vi "TWIN_v15_5.vi"() -> ()   [LabVIEW 2017]
uses:
  BERTTA/x64/Debug/BERTTA.dll
panel:
  in  "Add comment":string
  in  "OK Button":bool
  out "Started:":string
  in  "SHUTDOWN":bool
  in  "MASTER CONTROL":bool
  in  "Tab Control":T1(tab)
  out "Output File":path caption="selected path"
  in  "Browse folder":path=path "C:/Users/shresplab/Desktop" caption="start path"
  in  "Read Seq":bool
  in  "Save Seq":bool
  in  "Configuration file":path caption="Filename"
  in  "OK Button 2":bool
  out "Boolean":bool
  in  "User (initials)":string
  in  "Project name":string
  in  "Description":string
  out "Waveform Chart 9":dynamicdata(graph)
  out "Sensor OK 10":bool
  out "Sensor OK 9":bool
  out "Sensor OK 8":bool
  out "Sensor OK 7":bool
  out "Tr 2":dbl format="Tr:              %#_4g"
  out "Tj in 2":dbl format="Tj in:        %#_4g"
  out "Tj out 2":dbl format="Tj out:        %#_4g"
  out "T set 2":dbl format="T set:          %#_4g"
  out "Current step 3":i32 format="Current step:  %.0f"
  out "RPM 6":dbl format="RPM:          %#_g"
  out "Torque 4":dbl format="Torque:      %#_g"
  out "T external 5":dbl format="T (S2):       %#_4g"
  out "PUMP3 2":bool
  out "Led11 17":bool
  out "Target amount 2":dbl
  out "Scale weight 2":dbl
  out "Amount now 3":dbl
  out "Flow rate 2":dbl
  out "Time to target 5":dbl format="%<%H:%M:%S>t"
  out "Current step 2":dbl
  out "Target 2":dbl
  out "Amount now 2":dbl
  out "Led11 12":bool
  out "Target amount":dbl
  out "Scale weight":dbl
  out "Amount now":dbl
  out "Flow rate":dbl
  out "Time to target":dbl format="%<%H:%M:%S>t"
  out "Current step":dbl
  out "Target":dbl
  out "Amount now":dbl
  out "PUMP3":bool
  out "Led11 11":bool
  out "Amount now":dbl
  out "Target":dbl
  out "Current step":dbl
  out "Time to target":dbl format="%<%H:%M:%S>t"
  out "Flow rate":dbl
  out "Amount now":dbl
  out "Scale weight":dbl
  out "Target amount":dbl
  out "PUMP2":bool
  out "Target amount":dbl format="Target amount:        %#_g"
  out "Scale weight":dbl format="Scale weight:     %#_4g"
  out "Amount now":dbl format="Amount now:      %#_4g"
  out "Flow rate":dbl format="Flow rate:                   %#_4g"
  out "Time to target":dbl format="Time to target:     %<%H:%M:%S>t"
  out "Current step":dbl format="Current step:              %#_g"
  out "Target":dbl format="Target:                %#_4g"
  out "Amount now":dbl format="Amount now:    %#_4g"
  out "Led11 10":bool
  out "PUMP1":bool
  out "Sensor OK 6":bool
  out "Sensor OK 5":bool
  out "Sensor OK 4":bool
  out "Sensor OK 3":bool
  out "Tr":dbl format="Tr:              %#_4g"
  out "Tj in":dbl format="Tj in:        %#_4g"
  out "Tj out":dbl format="Tj out:        %#_4g"
  out "T set":dbl format="T set:          %#_4g"
  out "Current step":i32 format="Current step:  %.0f"
  out "RPM":dbl format="RPM:          %#_g"
  out "Torque 2":dbl format="Torque:      %#_g"
  out "T external 3":dbl format="T (S2):       %#_4g"
  out "Waveform Chart 5":dynamicdata(graph)
  out "Waveform Chart 6":dynamicdata(graph)
  out "Waveform Chart 7":dynamicdata(graph)
  in  "OK Button 11":bool=TRUE
  out "Table":string[][](table)=[["14.8.2017 18.06.59", "0,000000", "417,670000", "-0,150000", "1,000000", "22,220000", "23,366837", "23,574959", "23,985852", "23,690000", "240,000000", "4,000000", "0,000000", "397,000000", "-397,000000", "1,000000"], ["14.8.2017 18.07.06", "0,000000", "417,640000", "-0,120000", "1,000000", "22,220000", "23,763115", "23,906257", "23,985694", "23,680000", "240,000000", "4,000000", "0,000000", "397,000000", "-397,000000", "1,000000"], ["14.8.2017 18.07.13", "0,000000", "417,640000", "-0,120000", "1,000000", "22,220000", "23,965922", "24,013440", "23,984906", "23,670000", "240,000000", "4,100000", "3,000000", "397,000000", "-397,000000", "1,000000"], ["14.8.2017 18.07.21", "0,000000", "417,640000", "-0,120000", "1,000000", "22,220000", "23,943860", "23,900110", "23,987113", "23,670000", "240,000000", "4,000000", "0,000000", "397,000000", "-397,000000", "1,000000"], ["14.8.2017 18.07.28", "0,000000", "417,640000", "-0,120000", "1,000000", "22,220000", "23,736328", "23,600018", "23,989004", "23,660000", "240,000000", "4,000000", "0,000000", "397,000000", "-397,000000", "1,000000"], ["14.8.2017 18.07.36", "0,000000", "417,640000", "-0,120000", "1,000000", "22,220000", "23,480910", "23,324538", "23,991053", "23,660000", "240,000000", "4,000000", "0,000000", "397,000000", "-397,000000", "1,000000"], ["14.8.2017 18.07.43", "0,000000", "417,640000", "-0,120000", "2,000000", "22,220000", "23,195579", "23,008270", "23,999093", "23,650000", "240,000000", "4,000000", "0,000000", "397,000000", "-397,000000", "1,000000"], ["14.8.2017 18.07.51", "0,000000", "417,650000", "-417,650000", "1,000000", "22,220000", "22,862541", "22,649021", "24,003979", "23,650000", "240,000000", "4,000000", "0,000000", "397,000000", "-397,000000", "2,000000"], ["14.8.2017 18.07.58", "0,000000", "417,640000", "0,010000", "1,000000", "22,220000", "22,541353", "22,354878", "24,005398", "23,650000", "240,000000", "4,000000", "0,000000", "397,000000", "-397,000000", "1,000000"], ["14.8.2017 18.08.06", "0,000000", "417,640000", "0,010000", "1,000000", "22,220000", "22,347931", "22,253738", "24,007605", "23,640000", "240,000000", "4,100000", "0,000000", "397,000000", "-397,000000", "1,000000"], ["14.8.2017 18.08.13", "0,000000", "417,640000", "0,010000", "1,000000", "22,220000", "22,329030", "22,302102", "24,006028", "23,640000", "240,000000", "4,000000", "0,000000", "395,820000", "-395,820000", "1,000000"], ["14.8.2017 18.08.20", "0,000000", "417,640000", "0,010000", "1,000000", "22,220000", "22,466849", "22,511320", "24,002403", "23,630000", "240,000000", "4,000000", "0,000000", "395,830000", "-0,010000", "1,000000"], ["14.8.2017 18.08.28", "0,000000", "417,640000", "0,010000", "1,000000", "22,220000", "22,707062", "22,835101", "24,000984", "23,620000", "240,000000", "4,000000", "0,000000", "395,830000", "-0,010000", "1,000000"], ["14.8.2017 18.08.35", "0,000000", "417,640000", "0,010000", "1,000000", "22,220000", "23,054104", "23,232979", "24,001299", "23,600000", "240,000000", "4,000000", "0,000000", "395,830000", "-0,010000", "1,000000"], ["14.8.2017 18.08.43", "0,000000", "417,640000", "0,010000", "1,000000", "22,220000", "23,412371", "23,522793", "24,002560", "23,590000", "240,000000", "4,000000", "0,000000", "395,820000", "0,000000", "1,000000"], ["14.8.2017 18.08.51", "0,000000", "417,640000", "0,010000", "1,000000", "22,220000", "23,596247", "23,656125", "24,003821", "23,580000", "240,000000", "4,000000", "0,000000", "395,820000", "0,000000", "1,000000"]]
  out "LED_5 2":bool
  out "LED_4 2":bool
  in  "PAUSE/RUN 11":bool
  in  "TEMP RAMP 2":dbl[][](array[numeric])
  out "LED_3 2":bool
  out "LED_2 2":bool
  out "LED_1 2":bool
  out "LED_MANUAL 2":bool
  in  "Reset 9":bool
  in  "Manual/Ramp 2":bool=TRUE
  in  "Sensor selector 2":bool=TRUE
  in  "Tr/Tj mode selector 2":bool=TRUE
  out "LED STOP 2":bool
  in  "Failsafe 2":dbl=20.0 format="Failsafe temperature:            %#_g"
  out "Current temp 2":dbl format="Current temperature S1:       %#_4g"
  out "Sensor OK 2":bool
  out "T external 4":dbl format="Current temperature S2:       %#_4g"
  in  "OK Button 10":bool
  out "Waveform Chart 2":dynamicdata(graph)
  out "LED_5":bool
  out "LED_4":bool
  in  "PAUSE/RUN 4":bool
  in  "TEMP RAMP":dbl[][](array[numeric])
  out "LED_3":bool
  out "LED_2":bool
  out "LED_1":bool
  out "LED_MANUAL":bool
  in  "Reset 6":bool
  in  "Manual/Ramp":bool=TRUE
  in  "Sensor selector":bool=TRUE
  in  "Tr/Tj mode selector":bool=TRUE
  out "LED STOP":bool
  in  "Failsafe":dbl=20.0 format="Failsafe temperature:            %#_g"
  out "Current temp":dbl format="Current temperature S1:       %#_4g"
  out "Sensor OK":bool
  out "T external 2":dbl format="Current temperature S2:       %#_4g"
  in  "OK Button 3":bool
  out "Waveform Chart":dynamicdata(graph)
  in  "X scales":i64(slide)=50 scale=0.0..100.0
  out "Waveform Chart 19":dynamicdata(graph)
  in  "CLEAR":bool
  in  "ENABLE":bool=TRUE
  out "Led11 16":bool
  out "Led11 15":bool
  in  "PAUSE/RUN 12":bool
  in  "Tube select 4":u32(ring) items=["Big tube", "Double big tube", "Medium tube", "Small tube"]
  in  "Reset 10":bool
  out "Led11 14":bool
  in  "?":bool
  in  "Grams / min 4":dbl
  out "RPM 5":dbl format="%_4f"
  out "Flow rate (g/min) 4":dbl
  out "Scale reading 4":dbl
  out "Step amount now 4":dbl
  out "Total amount now 4":dbl
  out "Elapsed / step 4":dbl format="%<%H:%M:%S>t"
  out "Time to target 4":dbl format="%<%H:%M:%S>t"
  out "Led5 6":bool
  out "Led4 7":bool
  out "Led3 6":bool
  out "Led2 6":bool
  out "Led1 6":bool
  in  "PumpSeq 7":dbl[][](array[numeric])=[[0.0, 0.0, 0.0, 0.0, 0.0, 0.0, 0.0, 0.0, 0.0, 0.0], [0.0, 0.0, 0.0, 0.0, 0.0, 0.0, 0.0, 0.0, 0.0, 0.0], [0.0, 0.0, 0.0, 0.0, 0.0, 0.0, 0.0, 0.0, 0.0, 0.0], [0.0, 0.0, 0.0, 0.0, 0.0, 0.0, 0.0, 0.0, 0.0, 0.0], [0.0, 0.0, 0.0, 0.0, 0.0, 0.0, 0.0, 0.0, 0.0, 0.0], [0.0, 0.0, 0.0, 0.0, 0.0, 0.0, 0.0, 0.0, 0.0, 0.0], [0.0, 0.0, 0.0, 0.0, 0.0, 0.0, 0.0, 0.0, 0.0, 0.0], [0.0, 0.0, 0.0, 0.0, 0.0, 0.0, 0.0, 0.0, 0.0, 0.0], [0.0, 0.0, 0.0, 0.0, 0.0, 0.0, 0.0, 0.0, 0.0, 0.0], [0.0, 0.0, 0.0, 0.0, 0.0, 0.0, 0.0, 0.0, 0.0, 0.0]]
  out "Led11 13":bool
  in  "PAUSE/RUN 9":bool=TRUE
  out "Led11 7":bool
  out "Led11 6":bool
  in  "PAUSE/RUN 3":bool
  in  "Tube select 3":u32(ring) items=["Big tube", "Double big tube", "Medium tube", "Small tube"]
  in  "Reset 8":bool
  out "Led11 9":bool
  in  "?":bool
  in  "Grams / min 3":dbl
  out "RPM 3":dbl format="%_4f"
  out "Flow rate (g/min) 3":dbl
  out "Scale reading 3":dbl
  out "Step amount now 3":dbl
  out "Total amount now 3":dbl
  out "Elapsed / step 3":dbl format="%<%H:%M:%S>t"
  out "Time to target 3":dbl format="%<%H:%M:%S>t"
  out "Led5 5":bool
  out "Led4 5":bool
  out "Led3 5":bool
  out "Led2 5":bool
  out "Led1 5":bool
  in  "PumpSeq 6":dbl[][](array[numeric])=[[0.0, 0.0, 0.0, 0.0, 0.0, 0.0, 0.0, 0.0, 0.0, 0.0], [0.0, 0.0, 0.0, 0.0, 0.0, 0.0, 0.0, 0.0, 0.0, 0.0], [0.0, 0.0, 0.0, 0.0, 0.0, 0.0, 0.0, 0.0, 0.0, 0.0], [0.0, 0.0, 0.0, 0.0, 0.0, 0.0, 0.0, 0.0, 0.0, 0.0], [0.0, 0.0, 0.0, 0.0, 0.0, 0.0, 0.0, 0.0, 0.0, 0.0], [0.0, 0.0, 0.0, 0.0, 0.0, 0.0, 0.0, 0.0, 0.0, 0.0], [0.0, 0.0, 0.0, 0.0, 0.0, 0.0, 0.0, 0.0, 0.0, 0.0], [0.0, 0.0, 0.0, 0.0, 0.0, 0.0, 0.0, 0.0, 0.0, 0.0], [0.0, 0.0, 0.0, 0.0, 0.0, 0.0, 0.0, 0.0, 0.0, 0.0], [0.0, 0.0, 0.0, 0.0, 0.0, 0.0, 0.0, 0.0, 0.0, 0.0]]
  out "Led11 8":bool
  in  "PAUSE/RUN 8":bool=TRUE
  out "Led11 7":bool
  out "Led11 6":bool
  in  "PAUSE/RUN 2":bool
  in  "Tube select 2":u32(ring) items=["Big tube", "Double big tube", "Medium tube", "Small tube"]
  out "Led11 7":bool
  in  "?":bool
  in  "Grams / min 2":dbl
  out "RPM 2":dbl format="%_4f"
  out "Flow rate (g/min) 2":dbl
  out "Scale reading 2":dbl
  out "Step amount now 2":dbl
  out "Total amount now 2":dbl
  out "Elapsed / step 2":dbl format="%<%H:%M:%S>t"
  out "Time to target 2":dbl format="%<%H:%M:%S>t"
  out "Led5 4":bool
  out "Led4 4":bool
  out "Led3 4":bool
  out "Led2 4":bool
  out "Led1 4":bool
  in  "PumpSeq 5":dbl[][](array[numeric])=[[0.0, 0.0, 0.0, 0.0, 0.0, 0.0, 0.0, 0.0, 0.0, 0.0], [0.0, 0.0, 0.0, 0.0, 0.0, 0.0, 0.0, 0.0, 0.0, 0.0], [0.0, 0.0, 0.0, 0.0, 0.0, 0.0, 0.0, 0.0, 0.0, 0.0], [0.0, 0.0, 0.0, 0.0, 0.0, 0.0, 0.0, 0.0, 0.0, 0.0], [0.0, 0.0, 0.0, 0.0, 0.0, 0.0, 0.0, 0.0, 0.0, 0.0], [0.0, 0.0, 0.0, 0.0, 0.0, 0.0, 0.0, 0.0, 0.0, 0.0], [0.0, 0.0, 0.0, 0.0, 0.0, 0.0, 0.0, 0.0, 0.0, 0.0], [0.0, 0.0, 0.0, 0.0, 0.0, 0.0, 0.0, 0.0, 0.0, 0.0], [0.0, 0.0, 0.0, 0.0, 0.0, 0.0, 0.0, 0.0, 0.0, 0.0], [0.0, 0.0, 0.0, 0.0, 0.0, 0.0, 0.0, 0.0, 0.0, 0.0]]
  out "Led11 6":bool
  in  "Reset 7":bool
  in  "PAUSE/RUN 7":bool=TRUE
  out "Led5 7":bool
  out "Led4 6":bool
  in  "PAUSE/RUN":bool
  in  "Tube select":u32(ring) items=["Big tube", "Double big tube", "Medium tube", "Small tube"]
  out "Led11 5":bool
  out "RPM":dbl format="RPM                      %_4f"
  out "Flow rate (g/min)":dbl format="Flow rate               %#_g"
  out "Scale reading":dbl format="Scale reading       %#_g"
  out "Step amount now":dbl format="Step amount       %#_g"
  out "Total amount now":dbl format="Total amount      %#_g"
  out "Elapsed / step":dbl format="Elapsed / step      %<%H:%M:%S>t"
  out "Time to target":dbl format="Time to target     %<%H:%M:%S>t"
  out "Led5 3":bool
  out "Led4 3":bool
  out "Led3 3":bool
  out "Led2 3":bool
  out "Led1 3":bool
  in  "PumpSeq 4":dbl[][](array[numeric])=[[0.0, 0.0, 0.0, 0.0, 0.0, 0.0, 0.0, 0.0, 0.0, 0.0], [0.0, 0.0, 0.0, 0.0, 0.0, 0.0, 0.0, 0.0, 0.0, 0.0], [0.0, 0.0, 0.0, 0.0, 0.0, 0.0, 0.0, 0.0, 0.0, 0.0], [0.0, 0.0, 0.0, 0.0, 0.0, 0.0, 0.0, 0.0, 0.0, 0.0], [0.0, 0.0, 0.0, 0.0, 0.0, 0.0, 0.0, 0.0, 0.0, 0.0], [0.0, 0.0, 0.0, 0.0, 0.0, 0.0, 0.0, 0.0, 0.0, 0.0], [0.0, 0.0, 0.0, 0.0, 0.0, 0.0, 0.0, 0.0, 0.0, 0.0], [0.0, 0.0, 0.0, 0.0, 0.0, 0.0, 0.0, 0.0, 0.0, 0.0], [0.0, 0.0, 0.0, 0.0, 0.0, 0.0, 0.0, 0.0, 0.0, 0.0], [0.0, 0.0, 0.0, 0.0, 0.0, 0.0, 0.0, 0.0, 0.0, 0.0]]
  in  "?":bool
  in  "Grams / min":dbl format="Manual g/min:  %#_g"
  out "Led11 4":bool
  in  "Reset 5":bool
  out "Waveform Chart 18":dynamicdata(graph)
  in  "OK Button 4":bool
  out "Waveform Chart 16":dynamicdata(graph)
  in  "OK Button 5":bool
  out "Waveform Chart 17":dynamicdata(graph)
  in  "OK Button 6":bool
  in  "PAUSE/RUN 5":bool
  in  "?":bool
  in  "Scale port":dbl=5.0
  out "Waveform Chart 15":dynamicdata(graph)
  in  "OK Button 8":bool
  in  "PAUSE/RUN 10":bool
  in  "Set RPM 2":i32
  in  "Remote / Manual 2":bool
  out "RPM 4":dbl
  out "Torque 3":dbl
  out "Waveform Chart 8":dynamicdata(graph)
  in  "OK Button 9":bool
  in  "PAUSE/RUN 6":bool
  in  "Set RPM":i32
  in  "Remote / Manual":bool
  out "RPM":dbl
  out "Torque":dbl
  out "Waveform Chart 4":dynamicdata(graph)
  in  "OK Button 7":bool
  in  "CDAQ 1 Temp Control 2":tag="EASY9217_2"
  in  "PORT PUMP3 2":i32 format="PUMP 4 PORT:  %.0f"
  in  "SCALE 4":i32 format="SCALE 4 PORT:  %.0f"
  in  "HEIDOLPH 2":i32=3 format="HEIDOLPH 2 PORT:  %.0f"
  in  "LAUDA 2":i32=2 format="LAUDA 2 PORT:  %.0f"
  in  "CDAQ 1 Temp Control":tag="EASY9217_1"
  in  "CDAQ PAM Control":tag="EASY9747"
  in  "PORT PUMP2":i32 format="PUMP 2 PORT:  %.0f"
  in  "PORT PUMP3":i32 format="PUMP 3 PORT:  %.0f"
  in  "PORT PUMP1":i32 format="PUMP 1 PORT:  %.0f"
  in  "Save PortDev":bool
  in  "LAUDA":i32 format="LAUDA 1 PORT:  %.0f"
  in  "HEIDOLPH":i32 format="HEIDOLPH 1 PORT:  %.0f"
  in  "SCALE1":i32 format="SCALE 1 PORT:  %.0f"
  in  "SCALE2":i32 format="SCALE 2 PORT:  %.0f"
  in  "SCALE 3":i32 format="SCALE 3 PORT:  %.0f"
  # "Sensor:"
  # "Control:"
  # "Sensor:"
  # "Control:"
  # "PUMP & SCALE 4"
  # "STEP"
  # "TOTAL"
  # "PUMP & SCALE 3"
  # "STEP"
  # "TOTAL"
  # "PUMP & SCALE 2"
  # "STEP"
  # "TOTAL"
  # "PUMP & SCALE 1"
  # "STEP"
  # "TOTAL"
  # "MANUAL"
  # "RAMP"
  # "Temp Target       Time Target          Wait Time"
  # "STOP"
  # "MANUAL"
  # "RAMP"
  # "Temp Target       Time Target          Wait Time"
  # "STOP"
  # "g              min"
  # "g              min"
  # "g              min"
  # "g              min"
  # "PAM control"
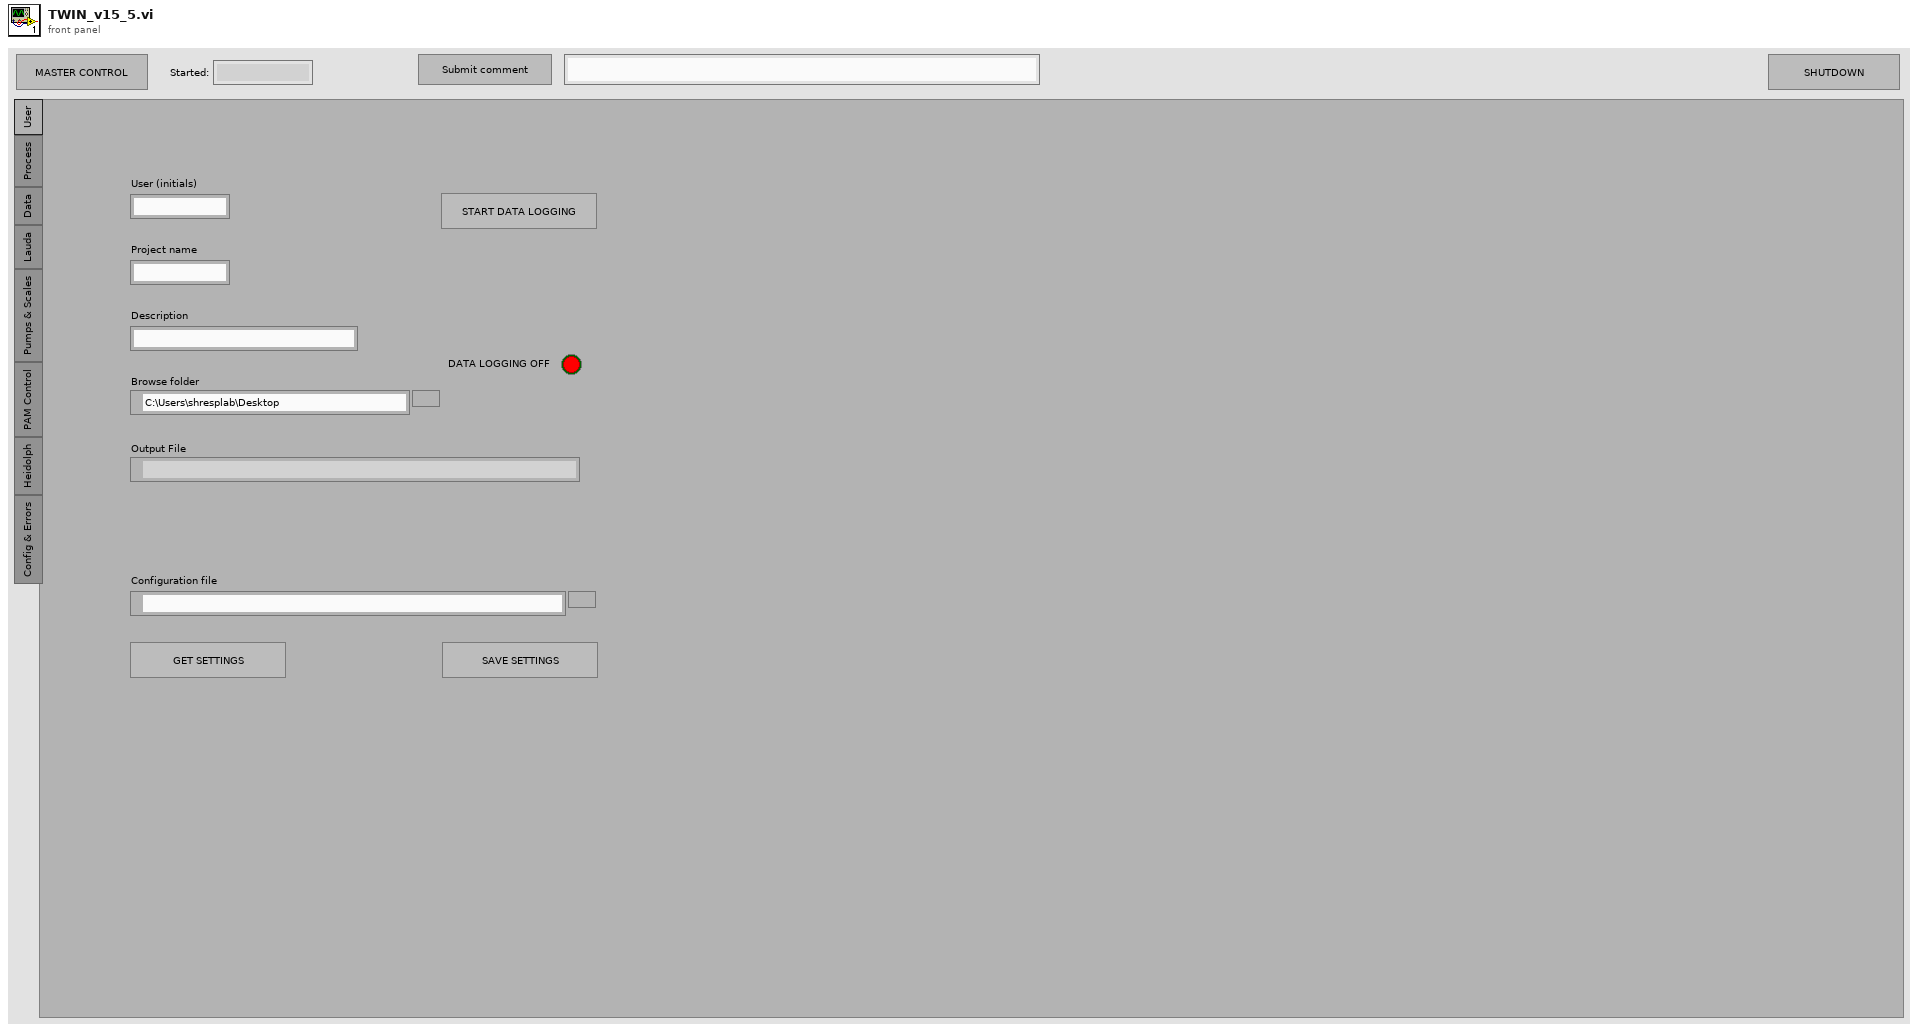
[diagram p1: front panel]
types:
  T1 = enum32{"User", "Process", "Data", "Lauda", "Pumps & Scales", "PAM Control", "Heidolph", "Config & Errors"}
diagram:
  n1 = while {
    i -> [w291]
    stop <- FALSE stop-if-true
    w225 = i64 1000 ("y")
    # "SCALE & PUMP 3"
    n2 = And(x="PAUSE/RUN 10", y="MASTER CONTROL") -> (x .and. y?=w75:bool)
    n3 = And(x="PAUSE/RUN 6", y="MASTER CONTROL") -> (x .and. y?=w215:bool)
    n4 = Not(x="MASTER CONTROL") -> (.not. x?=w326:bool)
    n5 = Boolean To (0,1)(Boolean="PAUSE/RUN 7") -> (0, 1=w4:i16)
    n6 = Boolean To (0,1)(Boolean="PAUSE/RUN 8") -> (0, 1=w3:i16)
    n7 = Boolean To (0,1)(Boolean="PAUSE/RUN 9") -> (0, 1=w2:i16)
    n8 = Boolean To (0,1)(Boolean="ENABLE") -> (0, 1=w1:i16)
    n9 = control-ref of="This VI"() -> (w211:refnum<vi>)
    n10 = Multiply(x="X scales", y=w225) -> (x*y=w226:i64)
    n11 = Boolean To (0,1)(Boolean=w326) -> (0, 1=w327:i16)
    n12 = call "RampCTRL_1.vi"("TEMP RAMP"="TEMP RAMP", "Reset 6"="Reset 6") -> ("Array"=w248:dbl[], "Array 2"=w249:dbl[], "Array 3"=w250:dbl[])  [unwired: 7 in]
    n13 = Add(x=w226, y=w225) -> (x+y=w63:i64)
    n14 = for {
      N: w327 -> [_]
      n15 = Get Date/Time String(want seconds? (F)=TRUE) -> (time string=→"Started:":string)  [unwired: 2 in, 1 out]
    }
    n16 = Select(t="Set RPM", s=w215, f=10) -> (s? t:f=w218:i32)
    n17 = Select(t="Set RPM 2", s=w75, f=10) -> (s? t:f=w72:i32)
    n18 = Boolean To (0,1)(Boolean="Sensor selector") -> (0, 1=w243:i16)
    n19 = feedback #1() -> (w224:i64)  [unwired: 1 in]
    n20 = feedback-in #1(w63) -> ()
    n21 = call "shutdown sequence.vi"("SHUTDOWN"="SHUTDOWN", "VI in"=w211) -> ()  [unwired: 10 in]
    n22 = Boolean To (0,1)(Boolean="SHUTDOWN") -> (0, 1=w210:i16)
    n23 = Boolean To (0,1)(Boolean="Reset 6") -> (0, 1=w260:i16)
    n24 = property on="Waveform Chart 2" class="WFChart (strict)"() -> ("History Data"=w65:dynamicdata[])  [unwired: 2 in, 2 out]
    n25 = Not Equal?(x=w224, y=w63) -> (x != y?=w223:bool)
    n26 = property on="Waveform Chart" class="WFChart (strict)"() -> ("History Data"=w228:dynamicdata[])  [unwired: 2 in, 2 out]
    n27 = Boolean To (0,1)(Boolean="SHUTDOWN") -> (0, 1=w212:i16)
    n28 = call "ReadMoxa12.vi"("PORT 1"="LAUDA", "PORT 2"="LAUDA 2", "PORT 3"="HEIDOLPH", "PORT 4"="HEIDOLPH 2", "PORT 5"="SCALE1", "PORT 6"="SCALE2", "PORT 7"="SCALE 3", "PORT 8"="SCALE 4", "enable1"=w4, "enable2"=w3, "enable3"=w2, "enable4"=w1) -> ("params"=w49:dbl[])  [unwired: 7 in]
    n29 = Boolean To (0,1)(Boolean=w223) -> (0, 1=w221:i16)
    n30 = Array Size(array=w228) -> (size(s)=w222:i32)
    n31 = Array Size(array=w65) -> (size(s)=w64:i32)
    n32 = call "HEI_CTRL.vi"("shutdown"=w212, "Set RPM"=w218, "Remote / Manual"="Remote / Manual", "port3"="HEIDOLPH") -> ()  [unwired: 8 in]
    n33 = Boolean To (0,1)(Boolean="Tr/Tj mode selector") -> (0, 1=w244:i16)
    n34 = call "SensorMode1.vi"("Numeric"=w243, "Numeric 2"=w244) -> ("Sensor OK 4"=→"Sensor OK 4":bool, "Sensor OK 5"=→"Sensor OK 5":bool, "Sensor OK 6"=→"Sensor OK 6":bool, "Sensor OK 3"=→"Sensor OK 3":bool)  [unwired: 6 in]
    n35 = for {
      N: w221 -> [_]
      tunnel: w222 -> [w346]
      tunnel: w63 -> [w345]
      tunnel: w64 -> [w342]
      tunnel: w63 -> [w341]
      n36 = Add(x=w342, y=w341) -> (x+y=w343:i64)
      n37 = Add(x=w346, y=w345) -> (x+y=w344:i64)
      n38 = property on="Waveform Chart" class="WFChart (strict)"("XScale.Maximum"=w344) -> ()  [unwired: 2 in, 2 out]
      n39 = property on="Waveform Chart 2" class="WFChart (strict)"("XScale.Maximum"=w343) -> ()  [unwired: 2 in, 2 out]
    }
    n40 = Boolean To (0,1)(Boolean="Manual/Ramp") -> (0, 1=w258:i16)
    n41 = And(x="MASTER CONTROL", y="PAUSE/RUN 4") -> (x .and. y?=w257:bool)
    n42 = Build Array("LAUDA", "LAUDA 2", "HEIDOLPH", "HEIDOLPH 2", "SCALE1", "SCALE2", "SCALE 3", "SCALE 4", "PORT PUMP1", "PORT PUMP2", "PORT PUMP3", "PORT PUMP3 2") -> (w232:i32[])
    n43 = Boolean To (0,1)(Boolean=w257) -> (0, 1=w256:i16)
    n44 = Boolean To (0,1)(Boolean="SHUTDOWN") -> (0, 1=w70:i16)
    n45 = call "LaudaDAQ.vi"("device name"="CDAQ 1 Temp Control") -> (1:"Tj out"=→"Tj out":dbl, "data"=w320:dynamicdata, "Sensor OK"=→"Sensor OK":bool, 4:"Tj out"=→"Tj in":dbl, "T external 2"=w214:dbl)  [unwired: 5 in, 1 out]
    "T external 2" <- w214
    "T external 3" <- w214
    n46 = call "Ramp_Lauda_v3.vi"("manual"=w258, "Tr_Tj"=w244, "shutdown"=w210, "S1_S2"=w243, "Tr"=w49, "T_fail"="Failsafe", "enable"=w256, "time_set"=w249, "reset"=w260, "time_wait"=w248, "T_S2"=w214, "port"="LAUDA", "T_sp"=w250) -> ("LED_1"=→"LED_1":bool, "LED_manual"=→"LED_MANUAL":bool, "LED_2"=→"LED_2":bool, "step"=w235:dbl, "LED_stop"=→"LED STOP":bool, "LED_3"=→"LED_3":bool, "LED 4"=→"LED_4":bool, "LED 5"=→"LED_5":bool, "setpoint"=w8:dbl, "Tr_out"=w255:dbl, "T int"=w254:dbl)  [unwired: 2 in, 2 out]
    "Tr" <- w255
    "T set" <- w8
    "Current temp" <- w255
    n47 = call "HEI_CTRL_2.vi"("shutdown"=w70, "Set RPM"=w72, "Remote / Manual"="Remote / Manual 2", "port3"="HEIDOLPH 2") -> ()  [unwired: 8 in]
    n48 = Boolean To (0,1)(Boolean="Save PortDev") -> (0, 1=w294:i16)
    n49 = for {
      N: w294 -> [_]
      tunnel: w232 -> [w400]
      tunnel: "Save PortDev" -> [w401]
      n50 = call "Convert to Dynamic Data"("Array"=w400) -> ("Dynamic Data Type"=w399:dynamicdata)  [unwired: 3 in]
      n51 = call "Write To Measurement File3"("Signals"=w399, "Reset"=w401) -> ()  [unwired: 15 in, 3 out]
    }
    n52 = Boolean To (0,1)(Boolean="OK Button 9") -> (0, 1=w67:i16)
    n53 = for {
      N: w67 -> [_]
      n54 = property on="Waveform Chart 8" class="WFChart (strict)"("History Data"=dynamicdata[] []) -> ()  [unwired: 2 in, 2 out]
    }
    n55 = Add(x=w235, y=1.0) -> (x+y=→"Current step":dbl)
    n56 = Merge Signals(w8, w255, w254, w320) -> (w22:dynamicdata)
    "Waveform Chart" <- w22
    "Waveform Chart 5" <- w22
    n57 = Less?(x=w291, y=1.0) -> (x < y?=w289:bool)
    n58 = call "HEI_Data.vi"("params"=w49) -> ("Waveform Chart 8"=→"Waveform Chart 8":dynamicdata, "RPM"=→"RPM":dbl, "Dynamic Data"=w44:dynamicdata, "RPM 2"=→"RPM":dbl, "RPM 6"=→"RPM 6":dbl, "Torque 4"=→"Torque 4":dbl, "Torque 2"=→"Torque 2":dbl, "Waveform Chart 4"=→"Waveform Chart 4":dynamicdata, "Torque 3"=→"Torque 3":dbl, "Torque"=→"Torque":dbl, "RPM 4"=→"RPM 4":dbl, "Waveform Chart 6"=→"Waveform Chart 6":dynamicdata)  [unwired: 7 in]
    n59 = Boolean To (0,1)(Boolean=w289) -> (0, 1=w290:i16)
    n60 = for {
      N: w290 -> [_]
      tunnel: w289 -> [w394]
      n61 = while {
        tunnel: [w397] -> w393
        tunnel: w394 -> [w395]
        stop <- w398 stop-if-true
        n62 = call "Read From Measurement File2"("Enable"=TRUE, "Reset"=w395) -> ("Signals"=w397:dynamicdata, "EOF?"=w398:bool)  [unwired: 4 in, 4 out]
      }
      n63 = call "Convert from Dynamic Data2"("Dynamic Data Type"=w393) -> ("Array"=w369:dbl[])  [unwired: 3 in]
      n64 = Index Array(array=w369, index=0) -> (element=w386:dbl)
      n65 = Index Array(array=w369, index=1) -> (element=w375:dbl)
      n66 = Index Array(array=w369, index=2) -> (element=w385:dbl)
      n67 = Index Array(array=w369, index=3) -> (element=w373:dbl)
      n68 = Index Array(array=w369, index=4) -> (element=w384:dbl)
      n69 = Index Array(array=w369, index=5) -> (element=w383:dbl)
      n70 = Index Array(array=w369, index=6) -> (element=w382:dbl)
      n71 = Index Array(array=w369, index=7) -> (element=w371:dbl)
      n72 = Index Array(array=w369, index=8) -> (element=w377:dbl)
      n73 = Index Array(array=w369, index=9) -> (element=w379:dbl)
      n74 = Index Array(array=w369, index=10) -> (element=w378:dbl)
      n75 = Index Array(array=w369, index=11) -> (element=w368:dbl)
      n76 = property on="LAUDA" class="DigNum (strict)"("Val(Sgnl)"=w386) -> ()  [unwired: 2 in, 2 out]
      n77 = property on="LAUDA 2" class="DigNum (strict)"("Val(Sgnl)"=w375) -> ()  [unwired: 2 in, 2 out]
      n78 = property on="HEIDOLPH" class="DigNum (strict)"("Val(Sgnl)"=w385) -> ()  [unwired: 2 in, 2 out]
      n79 = property on="HEIDOLPH 2" class="DigNum (strict)"("Val(Sgnl)"=w373) -> ()  [unwired: 2 in, 2 out]
      n80 = property on="SCALE1" class="DigNum (strict)"("Val(Sgnl)"=w384) -> ()  [unwired: 2 in, 2 out]
      n81 = property on="SCALE2" class="DigNum (strict)"("Val(Sgnl)"=w383) -> ()  [unwired: 2 in, 2 out]
      n82 = property on="SCALE 3" class="DigNum (strict)"("Val(Sgnl)"=w382) -> ()  [unwired: 2 in, 2 out]
      n83 = property on="SCALE 4" class="DigNum (strict)"("Val(Sgnl)"=w371) -> ()  [unwired: 2 in, 2 out]
      n84 = property on="PORT PUMP1" class="DigNum (strict)"("Val(Sgnl)"=w377) -> ()  [unwired: 2 in, 2 out]
      n85 = property on="PORT PUMP2" class="DigNum (strict)"("Val(Sgnl)"=w379) -> ()  [unwired: 2 in, 2 out]
      n86 = property on="PORT PUMP3" class="DigNum (strict)"("Val(Sgnl)"=w378) -> ()  [unwired: 2 in, 2 out]
      n87 = property on="PORT PUMP3 2" class="DigNum (strict)"("Val(Sgnl)"=w368) -> ()  [unwired: 2 in, 2 out]
    }
    n88 = Boolean To (0,1)(Boolean="OK Button 3") -> (0, 1=w301:i16)
    n89 = Boolean To (0,1)(Boolean="Reset 9") -> (0, 1=w117:i16)
    n90 = for {
      N: w301 -> [_]
      n91 = property on="Waveform Chart" class="WFChart (strict)"("History Data"=dynamicdata[] []) -> ()  [unwired: 2 in, 2 out]
    }
    n92 = call "RampCTRL_2.vi"("TEMP RAMP in"="TEMP RAMP 2", "Reset 9"="Reset 9") -> ("Array"=w109:dbl[], "Array 2"=w110:dbl[], "Array 3"=w111:dbl[])  [unwired: 7 in]
    n93 = And(x="MASTER CONTROL", y="PAUSE/RUN 11") -> (x .and. y?=w124:bool)
    n94 = Boolean To (0,1)(Boolean="Manual/Ramp 2") -> (0, 1=w120:i16)
    n95 = Boolean To (0,1)(Boolean="Tr/Tj mode selector 2") -> (0, 1=w62:i16)
    n96 = Boolean To (0,1)(Boolean="Sensor selector 2") -> (0, 1=w61:i16)
    n97 = call "SensorMode2.vi"("Numeric"=w61, "Numeric 2"=w62) -> ("Sensor OK 8"=→"Sensor OK 8":bool, "Sensor OK 10"=→"Sensor OK 10":bool, "Sensor OK 9"=→"Sensor OK 9":bool, "Sensor OK 7"=→"Sensor OK 7":bool)  [unwired: 6 in]
    n98 = Boolean To (0,1)(Boolean=w124) -> (0, 1=w123:i16)
    n99 = call "LaudaDAQ2.vi"("device name"="CDAQ 1 Temp Control 2") -> (1:"Tj out"=→"Tj out 2":dbl, "data"=w41:dynamicdata, "Sensor OK"=→"Sensor OK 2":bool, 4:"Tj out"=→"Tj in 2":dbl, "T external 2"=→"T external 4" →"T external 5":dbl)  [unwired: 5 in, 1 out]
    n100 = call "Ramp_Lauda_v3_2.vi"("manual"=w120, "Tr_Tj"=w62, "S1_S2"=w61, "Tr"=w49, "T_fail"="Failsafe 2", "enable"=w123, "time_set"=w110, "reset"=w117, "time_wait"=w109, "T_sp"=w111) -> ("LED_1"=→"LED_1 2":bool, "LED_manual"=→"LED_MANUAL 2":bool, "LED_2"=→"LED_2 2":bool, "step"=w115:dbl, "LED_stop"=→"LED STOP 2":bool, "LED_3"=→"LED_3 2":bool, "LED 4"=→"LED_4 2":bool, "LED 5"=→"LED_5 2":bool, "setpoint"=w7:dbl, "Tr_out"=w108:dbl, "T int"=w107:dbl)  [unwired: 5 in, 2 out]
    "Current temp 2" <- w108
    "T set 2" <- w7
    "Tr 2" <- w108
    n101 = Boolean To (0,1)(Boolean="OK Button 4") -> (0, 1=w299:i16)
    n102 = Add(x=w115, y=1.0) -> (x+y=→"Current step 3":dbl)
    n103 = for {
      N: w299 -> [_]
      n104 = property on="Waveform Chart 18" class="WFChart (strict)"("History Data"=dynamicdata[] []) -> ()  [unwired: 2 in, 2 out]
    }
    n105 = Merge Signals(w7, w108, w107, w41) -> (w21:dynamicdata)
    "Waveform Chart 2" <- w21
    "Waveform Chart 9" <- w21
    n106 = Boolean To (0,1)(Boolean="OK Button 5") -> (0, 1=w241:i16)
    n107 = for {
      N: w241 -> [_]
      n108 = property on="Waveform Chart 16" class="WFChart (strict)"("History Data"=dynamicdata[] []) -> ()  [unwired: 2 in, 2 out]
    }
    n109 = call "IsmaCTRL.vi"("FR_manual"="Grams / min", "tube selector"="Tube select", "Manual"="?", "Reset"="Reset 5", "Pause"="PAUSE/RUN", "Setpoint_W   /   Setpoint_T"="PumpSeq 4", "Enable"="MASTER CONTROL", "Scale"=w49) -> ("Boolean 9"=→"Led11 5" →"Led11 10":bool, "Boolean"=→"Led1 3":bool, "Boolean 2"=→"Led2 3":bool, "Total target"=→"Target":dbl, "Boolean 3"=→"Led3 3":bool, "Boolean 4"=→"Led4 3":bool, "lastAmount"=→"Step amount now":dbl, "step"=→"Current step":dbl, "Boolean 5"=→"Led5 3":bool, "Boolean 6"=→"Led4 6":bool, "Boolean 7"=→"Led5 7":bool, "FR"=w193:dbl, "RPM"=w47:dbl, "Weight"=w189:dbl, "elapsed"=→"Elapsed / step":dbl, "time_to_target"=→"Time to target" →"Time to target":dbl, "pumpCTRL"=w205:dbl, "Target_step"=→"Target amount":dbl, "Boolean 8"=w197:bool)  [unwired: 1 out]
    "Flow rate" <- w193
    "Scale weight" <- w189
    "Led11 4" <- w197
    "Scale reading" <- w189
    "Flow rate (g/min)" <- w193
    "RPM" <- w47
    n110 = Boolean To (0,1)(Boolean="OK Button 6") -> (0, 1=w239:i16)
    n111 = for {
      N: w239 -> [_]
      n112 = property on="Waveform Chart 17" class="WFChart (strict)"("History Data"=dynamicdata[] []) -> ()  [unwired: 2 in, 2 out]
    }
    n113 = Multiply(x=w189, y=-1.0 ("x")) -> (x*y=→"Amount now" →"Amount now" →"Total amount now":dbl)
    n114 = And(x="PAUSE/RUN", y=w197) -> (x .and. y?=w277:bool)
    n115 = feedback #2() -> (w278:bool)  [unwired: 1 in]
    n116 = feedback-in #2(w277) -> ()
    n117 = Greater?(x=w205, y=70.0) -> (0:→"PUMP1":bool)
    n118 = Not Equal?(x=w278, y=w277) -> (x != y?=w276:bool)
    n119 = Boolean To (0,1)(Boolean=w276) -> (0, 1=w275:i16)
    n120 = for {
      N: w275 -> [_]
      n121 = property on="PAUSE/RUN" class="Bool (strict)"("Val(Sgnl)"=FALSE ("Value (Signaling)")) -> ()  [unwired: 2 in, 2 out]
    }
    n122 = Merge Signals(w189, w193) -> (w242:dynamicdata)
    "Waveform Chart 18" <- w242
    n123 = Boolean To (0,1)(Boolean="OK Button 7") -> (0, 1=w297:i16)
    n124 = for {
      N: w297 -> [_]
      n125 = property on="Waveform Chart 4" class="WFChart (strict)"("History Data"=dynamicdata[] []) -> ()  [unwired: 2 in, 2 out]
    }
    n126 = call "IsmaCTRL_2.vi"("FR_manual"="Grams / min 2", "tube selector"="Tube select 2", "Manual"="?", "Reset"="Reset 7", "Pause"="PAUSE/RUN 2", "Setpoint_W   /   Setpoint_T"="PumpSeq 5", "Enable"="MASTER CONTROL", "Scale"=w49) -> ("Boolean 9"=→"Led11 7" →"Led11 11":bool, "Boolean"=→"Led1 4":bool, "Boolean 2"=→"Led2 4":bool, "Total target"=→"Target":dbl, "Boolean 3"=→"Led3 4":bool, "Boolean 4"=→"Led4 4":bool, "lastAmount"=→"Amount now" →"Step amount now 2":dbl, "step"=→"Current step":dbl, "Boolean 5"=→"Led5 4":bool, "Boolean 6"=→"Led11 6":bool, "Boolean 7"=→"Led11 7":bool, "FR"=w176:dbl, "RPM"=w46:dbl, "Weight"=w177:dbl, "elapsed"=→"Elapsed / step 2":dbl, "time_to_target"=→"Time to target" →"Time to target 2":dbl, "pumpCTRL"=w170:dbl, "Target_step"=→"Target amount":dbl, "Boolean 8"=w160:bool)  [unwired: 1 out]
    "Scale weight" <- w177
    "Flow rate" <- w176
    "Led11 6" <- w160
    "Scale reading 2" <- w177
    "Flow rate (g/min) 2" <- w176
    "RPM 2" <- w46
    n127 = Boolean To (0,1)(Boolean="OK Button 8") -> (0, 1=w284:i16)
    n128 = for {
      N: w284 -> [_]
      n129 = property on="Waveform Chart 15" class="WFChart (strict)"("History Data"=dynamicdata[] []) -> ()  [unwired: 2 in, 2 out]
    }
    n130 = Merge Signals(w177, w176) -> (w272:dynamicdata)
    "Waveform Chart 16" <- w272
    n131 = Multiply(x=w177, y=-1.0) -> (x*y=→"Amount now" →"Total amount now 2":dbl)
    n132 = And(x="PAUSE/RUN 2", y=w160) -> (x .and. y?=w270:bool)
    n133 = Greater?(x=w170, y=70.0) -> (0:→"PUMP2":bool)
    n134 = feedback #3() -> (w271:bool)  [unwired: 1 in]
    n135 = feedback-in #3(w270) -> ()
    n136 = Not Equal?(x=w271, y=w270) -> (x != y?=w269:bool)
    n137 = Boolean To (0,1)(Boolean=w269) -> (0, 1=w268:i16)
    n138 = for {
      N: w268 -> [_]
      n139 = property on="PAUSE/RUN 2" class="Bool (strict)"("Val(Sgnl)"=FALSE ("Value (Signaling)")) -> ()  [unwired: 2 in, 2 out]
    }
    n140 = Boolean To (0,1)(Boolean="CLEAR") -> (0, 1=w77:i16)
    n141 = for {
      N: w77 -> [_]
      n142 = property on="Waveform Chart 19" class="WFChart (strict)"("History Data"=dynamicdata[] []) -> ()  [unwired: 2 in, 2 out]
    }
    n143 = call "IsmaCTRL_3.vi"("FR_manual"="Grams / min 3", "tube selector"="Tube select 3", "Manual"="?", "Reset"="Reset 8", "Pause"="PAUSE/RUN 3", "Setpoint_W   /   Setpoint_T"="PumpSeq 6", "Enable"="MASTER CONTROL", "Scale"=w49) -> ("Boolean 9"=→"Led11 9" →"Led11 12":bool, "Boolean"=→"Led1 5":bool, "Boolean 2"=→"Led2 5":bool, "Total target"=→"Target":dbl, "Boolean 3"=→"Led3 5":bool, "Boolean 4"=→"Led4 5":bool, "lastAmount"=→"Amount now" →"Step amount now 3":dbl, "step"=→"Current step":dbl, "Boolean 5"=→"Led5 5":bool, "Boolean 6"=→"Led11 6":bool, "Boolean 7"=→"Led11 7":bool, "FR"=w146:dbl, "RPM"=w45:dbl, "Weight"=w145:dbl, "elapsed"=→"Elapsed / step 3":dbl, "time_to_target"=→"Time to target" →"Time to target 3":dbl, "pumpCTRL"=w151:dbl, "Target_step"=→"Target amount":dbl, "Boolean 8"=w136:bool)  [unwired: 1 out]
    "Scale weight" <- w145
    "Flow rate" <- w146
    "Led11 8" <- w136
    "Scale reading 3" <- w145
    "Flow rate (g/min) 3" <- w146
    "RPM 3" <- w45
    n144 = Multiply(x=w145, y=-1.0) -> (x*y=→"Amount now" →"Total amount now 3":dbl)
    n145 = Merge Signals(w189, w177, w145) -> (→"Waveform Chart 7":dynamicdata)
    n146 = Greater?(x=w151, y=70.0) -> (0:→"PUMP3":bool)
    n147 = And(x="MASTER CONTROL", y=w136) -> (x .and. y?=w263:bool)
    n148 = Merge Signals(w145, w146) -> (w265:dynamicdata)
    "Waveform Chart 17" <- w265
    n149 = feedback #4() -> (w264:bool)  [unwired: 1 in]
    n150 = feedback-in #4(w263) -> ()
    n151 = Not Equal?(x=w264, y=w263) -> (x != y?=w262:bool)
    n152 = Boolean To (0,1)(Boolean=w262) -> (0, 1=w261:i16)
    n153 = for {
      N: w261 -> [_]
      n154 = property on="PAUSE/RUN 3" class="Bool (strict)"("Val(Sgnl)"=FALSE ("Value (Signaling)")) -> ()  [unwired: 2 in, 2 out]
    }
    n155 = call "Convert to Dynamic Data6"("2D Array"="PumpSeq 7") -> ("Dynamic Data Type"=w10:dynamicdata)  [unwired: 3 in]
    n156 = call "Convert to Dynamic Data4"("2D Array"="PumpSeq 6") -> ("Dynamic Data Type"=w307:dynamicdata)  [unwired: 3 in]
    n157 = call "Convert to Dynamic Data3"("2D Array"="PumpSeq 5") -> ("Dynamic Data Type"=w308:dynamicdata)  [unwired: 3 in]
    n158 = call "Convert to Dynamic Data2"("2D Array"="PumpSeq 4") -> ("Dynamic Data Type"=w310:dynamicdata)  [unwired: 3 in]
    n159 = Merge Signals(w10, w307, w308, w310) -> (w309:dynamicdata)
    n160 = call "IsmaCTRL_4.vi"("FR_manual"="Grams / min 4", "tube selector"="Tube select 4", "Manual"="?", "Reset"="Reset 10", "Pause"="PAUSE/RUN 12", "Setpoint_W   /   Setpoint_T"="PumpSeq 7", "Enable"="MASTER CONTROL") -> ("Boolean 9"=→"Led11 14" →"Led11 17":bool, "Boolean"=→"Led1 6":bool, "Boolean 2"=→"Led2 6":bool, "Total target"=→"Target 2":dbl, "Boolean 3"=→"Led3 6":bool, "Boolean 4"=→"Led4 7":bool, "lastAmount"=→"Step amount now 4" →"Amount now 3":dbl, "step"=→"Current step 2":dbl, "Boolean 5"=→"Led5 6":bool, "Boolean 6"=→"Led11 15":bool, "Boolean 7"=→"Led11 16":bool, "FR"=w35:dbl, "RPM"=w43:dbl, "Weight"=w78:dbl, "elapsed"=→"Elapsed / step 4":dbl, "time_to_target"=→"Time to target 4" →"Time to target 5":dbl, "pumpCTRL"=w86:dbl, "Target_step"=→"Target amount 2":dbl, "Boolean 8"=w95:bool)  [unwired: 1 in, 1 out]
    "Led11 13" <- w95
    "Scale reading 4" <- w78
    "Flow rate (g/min) 4" <- w35
    "RPM 5" <- w43
    "Flow rate 2" <- w35
    "Scale weight 2" <- w78
    n161 = call "WriteMoxa12.vi"("PORT LAUDA 1"="LAUDA", "DATA LAUDA 1"=w8, "enable2"=w3, "DATA LAUDA 2"=w7, "DATA ISMA 1"=w47, "PORT LAUDA 2"="LAUDA 2", "DATA ISMA 2"=w46, "enable1"=w4, "enable4"=w1, "PORT ISMA 1"="PORT PUMP1", "DATA ISMA 3"=w45, "PORT ISMA 2"="PORT PUMP2", "PORT ISMA 3"="PORT PUMP3", "PORT ISMA 4"="PORT PUMP3 2", "enable3"=w2, "DATA ISMA 4"=w43) -> ()
    n162 = Boolean To (0,1)(Boolean="Save Seq") -> (0, 1=w306:i16)
    n163 = for {
      N: w306 -> [_]
      tunnel: w309 -> [w436]
      tunnel: "Configuration file" -> [w437]
      tunnel: "Save Seq" -> [w435]
      n164 = call "Write To Measurement File2"("Signals"=w436, "Reset"=w435, "Filename"=w437) -> ()  [unwired: 14 in, 3 out]
    }
    n165 = Multiply(x=w78, y=-1.0) -> (x*y=w79:dbl)
    "Total amount now 4" <- w79
    "Amount now 2" <- w79
    n166 = Greater?(x=w86, y=70.0) -> (0:→"PUMP3 2":bool)
    n167 = And(x="MASTER CONTROL", y=w95) -> (x .and. y?=w98:bool)
    n168 = feedback #5() -> (w99:bool)  [unwired: 1 in]
    n169 = feedback-in #5(w98) -> ()
    n170 = Merge Signals(w79, w35) -> (w23:dynamicdata)
    "Waveform Chart 19" <- w23
    n171 = Not Equal?(x=w99, y=w98) -> (x != y?=w97:bool)
    n172 = Boolean To (0,1)(Boolean=w97) -> (0, 1=w96:i16)
    n173 = for {
      N: w96 -> [_]
      n174 = property on="PAUSE/RUN 12" class="Bool (strict)"("Val(Sgnl)"=FALSE ("Value (Signaling)")) -> ()  [unwired: 2 in, 2 out]
    }
    n175 = Boolean To (0,1)(Boolean="Read Seq") -> (0, 1=w305:i16)
    n176 = for {
      N: w305 -> [_]
      tunnel: "Configuration file" -> [w420]
      tunnel: "Read Seq" -> [w419]
      n177 = while {
        tunnel: [w434] -> w430
        tunnel: w420 -> [w433]
        tunnel: w419 -> [w431]
        stop <- w432 stop-if-true
        n178 = call "Read From Measurement File"("Filename"=w433, "Reset"=w431) -> ("Signals"=w434:dynamicdata, "EOF?"=w432:bool)  [unwired: 4 in, 4 out]
      }
      n179 = call "Convert from Dynamic Data"("Dynamic Data Type"=w430) -> ("Array"=w423:dbl[][])  [unwired: 3 in]
      n180 = Array Subset(array=w423, index (row)=20 ("index"), length (row)=10 ("length")) -> (w416:dbl[][])  [unwired: 2 in]
      n181 = Array Subset(array=w423, index (row)=10 ("index"), length (row)=10 ("length")) -> (w417:dbl[][])  [unwired: 2 in]
      n182 = Array Subset(array=w423, index (row)=0 ("index"), length (row)=10 ("length")) -> (w415:dbl[][])  [unwired: 2 in]
      n183 = Array Subset(array=w423, index (row)=30 ("index"), length (row)=8 ("length")) -> (w418:dbl[][])  [unwired: 2 in]
      n184 = property on="PumpSeq 6" class="Arr (strict)"("Val(Sgnl)"=w417) -> ()  [unwired: 2 in, 2 out]
      n185 = property on="PumpSeq 7" class="Arr (strict)"("Val(Sgnl)"=w415) -> ()  [unwired: 2 in, 2 out]
      n186 = property on="PumpSeq 4" class="Arr (strict)"("Val(Sgnl)"=w418) -> ()  [unwired: 2 in, 2 out]
      n187 = property on="PumpSeq 5" class="Arr (strict)"("Val(Sgnl)"=w416) -> ()  [unwired: 2 in, 2 out]
    }
    n188 = Merge Signals(w242, w272, w265, w23) -> (w321:dynamicdata)
    n189 = Merge Signals(w22, w21, w321, w44) -> (w287:dynamicdata)
    n190 = Boolean To (0,1)(Boolean="OK Button 11") -> (0, 1=w5:i16)
    n191 = for {
      N: w5 -> [_]
      tunnel: w287 -> [w332]
      n192 = call "Build Table"("Include time data"=TRUE, "Signals"=w332) -> ("Table"=w336:string[][])  [unwired: 3 in, 6 out]
      n193 = Delete From Array(array=w336, length=23, index (col)=0 ("index (row)")) -> (array with subset deleted=→"Table":string[][])  [unwired: 1 in, 1 out]
    }
    n194 = Boolean To (0,1)(Boolean="PAUSE/RUN 5") -> (0, 1=w246:i16)
    n195 = for {
      N: w246 -> [_]
      tunnel: "MASTER CONTROL" -> [w350]
      tunnel: "PAUSE/RUN 5" -> [w349]
      n196 = And(x=w349, y="?") -> (x .and. y?=w358:bool)
      n197 = dll-call lib="C:/Users/shresplab/OneDrive - Kemira Oyj/Documents/GitHub/Bertta/BERTTA/x64/Debug/BERTTA.dll" fn="mettler"("port"="Scale port", "msg"=1) -> ("return type"=w352:dbl)  [unwired: 5 in, 2 out]
      n198 = And(x=w350, y=w358) -> (x .and. y?=w355:bool)
      n199 = Initialize Array(FALSE, 1 ("dimension size")) -> (w357:bool[])
      n200 = Replace Array Subset(array=w357, new element=w355, index=0) -> (w354:bool[])
      n201 = call "Convert to Dynamic Data5"("Double"=w352) -> ("Dynamic Data Type"=→"Waveform Chart 15":dynamicdata)  [unwired: 3 in]
      n202 = call "DAQ Assistant"("data"=w354, "device name"="CDAQ PAM Control") -> ()  [unwired: 16 in, 2 out]
    }
    n203 = call "filenameparser_09.vi"("Description"="Description", "start path"="Browse folder", "Project name"="Project name", "User (initials)"="User (initials)", "OK Button in"="OK Button 2") -> ("appended path 2"=w295:path, "appended path"=w323:path)  [unwired: 4 in, 1 out]
    "Output File" <- w295
    n204 = Boolean To (0,1)(Boolean="OK Button") -> (0, 1=w322:i16)
    n205 = for {
      N: w322 -> [_]
      tunnel: w323 -> [w407]
      w411 = " " ("string")
      n206 = property on="Add comment" class="Str"("Val(Sgnl)"="" ("Value (Signaling)")) -> ()  [unwired: 2 in, 2 out]
      n207 = Get Date/Time String(want seconds? (F)=TRUE) -> (date string=w414:string, time string=w412:string)  [unwired: 2 in]
      n208 = Concatenate Strings(w414, w411, w412, w411, "Add comment") -> (w410:string)
      n209 = feedback #6() -> (w409:string[])  [unwired: 1 in]
      n210 = Build Array (concatenate)(w409, w410) -> (w408:string[])
      n211 = feedback-in #6(w408) -> ()
      n212 = Write to Text File(file (use dialog)=w407, text=w408) -> ()  [unwired: 2 in, 3 out]
    }
    n213 = call "Header Names TWIN.vi"("Dynamic Data"=w287) -> ("Signals Out"=w288:dynamicdata)  [unwired: 10 in]
    n214 = call "Write To Measurement File"("Signals"=w288, "Enable"="OK Button 2", "Filename"=w295) -> ()  [unwired: 14 in, 3 out]
    "Boolean" <- "OK Button 2"
  }
